vi "String to option.vi"(11 "String in":string) -> (3 "String out":string)   [LabVIEW 2015]
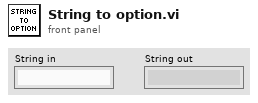
[diagram p1: front panel]
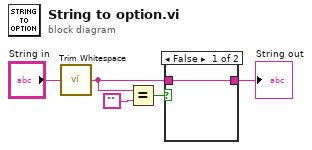
[diagram p0: block diagram]
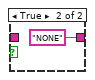
[diagram p2: hidden frame]
diagram:
  n1 = call <vilib>:"Trim Whitespace.vi"("string"="String in") -> ("trimmed string"=w5:string)  [unwired: 1 in]
  n2 = Equal?(x=w5, y="") -> (x = y?=w2:bool)
  n3 = case shown="False" w2 {
    tunnel: [w6 "NONE"] -> w4
    tunnel: w5 -> [w6 _]
    frame False {
    }
    frame True {
    }
  }
  "String out" <- w4
